vi "myRIO v1.0 ISR Worker.vi"   [LabVIEW 2021]
uses:
  <vilib>/myRIO/Common/Instrument Driver Framework/Utilities/typedefs/FPGA Ref Manager Action Enum.ctl
  <vilib>/Utility/error.llb/Error Cluster From Error Code.vi
  <vilib>/RVI Host/nirviSupport.llb/nirviErrorClusterFromErrorCode.vi
  <vilib>/rvi/errors/niLvFpgaAdjustHostInterfaceError.vi
  <vilib>/rvi/interface/nirviMethod/nirviMethod.xnode
  <vilib>/myRIO/Common/Instrument Driver Framework/Utilities/typedefs/Generic FPGA Reference.ctl
  <vilib>/rvi/interface/nirviMethod/StockFPGA_InlinedMethodWaitForMultipleIRQ.vi
  <vilib>/FPGAPlugInAG/Dynamic/niLvFpga_WaitOnIrq_Dynamic.vi
  <vilib>/FPGAPlugInAG/Dynamic/niLvFpga_AcknowledgeIrq_Dynamic.vi
types:
  T1 = typedef "FPGA Ref Manager Action Enum.ctl" = enum16{"Get", "Set", "Reset"}
  T2 = typedef "Generic FPGA Reference.ctl" = refnum<k20>
  T3 = typedef "Generic IRQ Array.ctl" = T4[]
  T4 = typedef "Generic IRQ.ctl" = cluster{"IRQ Type":T5, "IO IRQ Channels Enum":T6, "Callback VI Ref":T7, "Allow Overwrite?":bool, "Interrupt enabled?":bool}
  T5 = typedef "IRQ Type.ctl" = enum16{"Timer", "Analog falling edge", "Analog rising edge", "Digital falling edge", "Digital rising edge", "Digital edge"}
  T6 = typedef "IO IRQ Channels Enum.ctl" = enum16{"Not Connected", "A/AI0 (Interrupt)", "A/AI1 (Interrupt)", "A/DIO0 (Interrupt)", "A/DIO1 (Interrupt)", "A/DIO2 (Interrupt)", "A/DIO3 (Interrupt)", "Button0 (Interrupt)", "B/AI0 (Interrupt)", "B/AI1 (Interrupt)", "B/DIO0 (Interrupt)", "B/DIO1 (Interrupt)", "B/DIO2 (Interrupt)", "B/DIO3 (Interrupt)"}
  T7 = typedef "Callback VI Ref.ctl" = refnum<vi>
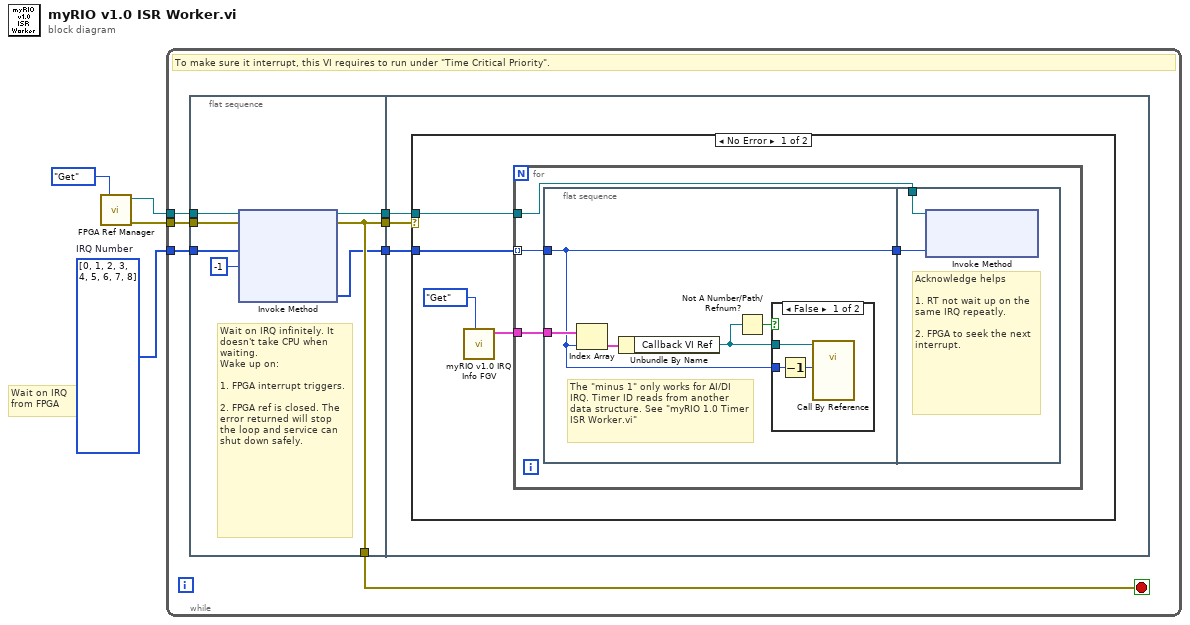
[diagram p0: block diagram]
diagram:
  w4 = i32[] [0, 1, 2, 3, 4, 5, 6, 7, 8]  # IRQ Number
  # "Wait on IRQ \nfrom FPGA"
  n1 = call <vilib>:"FPGA Ref Manager.vi"("Action"=FPGA_Ref_Manager_Action_Enum."Get") -> ("error out"=w1:errorcluster, "Generic FPGA Reference out"=w2:T2)  [unwired: 8 in]
  n2 = while {
    tunnel: w4 -> [w9]
    tunnel: w2 -> [w6]
    tunnel: w1 -> [w5]
    stop <- w10 stop-if-true
    # "To make sure it interrupt, this VI requires to run under \"Time Critical Priority\"."
    n3 = flat-sequence {
      tunnel: [w17] -> w11
      tunnel: [w15] -> w10
      tunnel: w9 -> [w16]
      tunnel: [w14] -> w8
      tunnel: [w15] -> w7
      tunnel: w6 -> [w13]
      tunnel: w5 -> [w12]
      tunnel: w11 -> [w21]
      tunnel: w8 -> [w20]
      tunnel: w7 -> [w19]
      frame #0 {
        # "Wait on IRQ infinitely. It doesn't take CPU when waiting.\nWake up on:\n\n1. FPGA interrupt triggers.\n\n2. FPGA ref is closed. The error returned will stop the loop and service can shut down safely."
        n4 = xnode "Invoke Method"("FPGA VI Reference In"=w13, "error in"=w12, "IRQ Number(s)"=w16, "Timeout (ms)"=-1) -> ("FPGA VI Reference Out"=w17:T2, "error out"=w15:errorcluster, "IRQ(s) Asserted"=w14:i32[])  [unwired: 1 out]
      }
      frame #1 {
        n5 = case shown="No Error" w19 {
          tunnel: w21 -> [w25 _]
          tunnel: w20 -> [w24 _]
          frame No Error {
            n6 = call <vilib>:"myRIO v1.0 IRQ Info FGV.vi"("Action"=FPGA_Ref_Manager_Action_Enum."Get") -> ("Generic IRQ Info out"=w22:T3)  [unwired: 9 in, 1 out]
            n7 = for {
              tunnel: w25 -> [w27]
              tunnel: w24 -> [w28] mode=indexing
              tunnel: w22 -> [w29]
              n8 = flat-sequence {
                tunnel: w29 -> [w34]
                tunnel: w28 -> [w30]
                tunnel: [w30] -> w26
                tunnel: w27 -> [w39]
                tunnel: w26 -> [w38]
                frame #0 {
                  # "The \"minus 1\" only works for AI/DI IRQ. Timer ID reads from another data structure. See \"myRIO 1.0 Timer ISR Worker.vi\""
                  n9 = Index Array(array=w34, index=w30) -> (element=w33:T4)
                  n10 = Unbundle By Name(w33) -> ("Callback VI Ref"=w32:T7)
                  n11 = Not A Number/Path/Refnum?(number/path/refnum=w32) -> (NaN/Path/Refnum?=w31:bool)
                  n12 = case shown="False" w31 {
                    tunnel: w32 -> [w36 _]
                    tunnel: w30 -> [w37 _]
                    frame False {
                      n13 = Decrement(x=w37) -> (x-1=w35:i32)
                      n14 = call-by-ref "?"(reference=w36, "ID"=w35) -> ()  [unwired: 12 in, 2 out]
                    }
                    frame True {
                    }
                  }
                }
                frame #1 {
                  # "Acknowledge helps \n\n1. RT not wait up on the same IRQ repeatly.\n\n2. FPGA to seek the next interrupt."
                  n15 = xnode "Invoke Method"("FPGA VI Reference In"=w39, "IRQ Number(s)"=w38) -> ()  [unwired: 1 in, 2 out]
                }
              }
            }
          }
          frame Error {
          }
        }
      }
    }
  }
